vi "eFGV - Stop RT.vi"(6 "State":T1, 8 "error in (no error)":errorcluster, 10 "Stop RT":bool) -> (0 "error out":errorcluster, 2 "Stop RT Event":refnum<user-event>)   [LabVIEW 2020]
uses:
  Shared/Control/State - eFGV.ctl
  <vilib>/event_ctls.llb/usereventprio.ctl
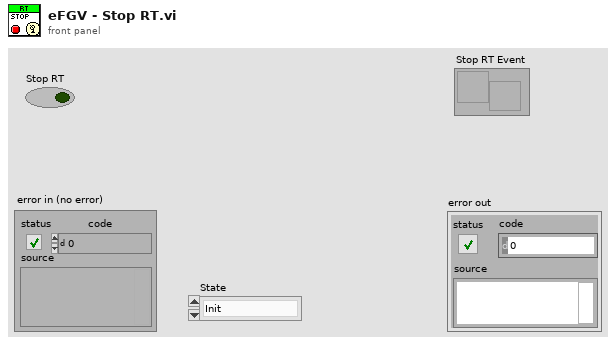
[diagram p1: front panel]
types:
  T1 = typedef "State - eFGV.ctl" = enum16{"Init", "Read", "Write", "Close"}
  T2 = typedef "usereventprio.ctl" = enum32{"high priority", "normal priority"}
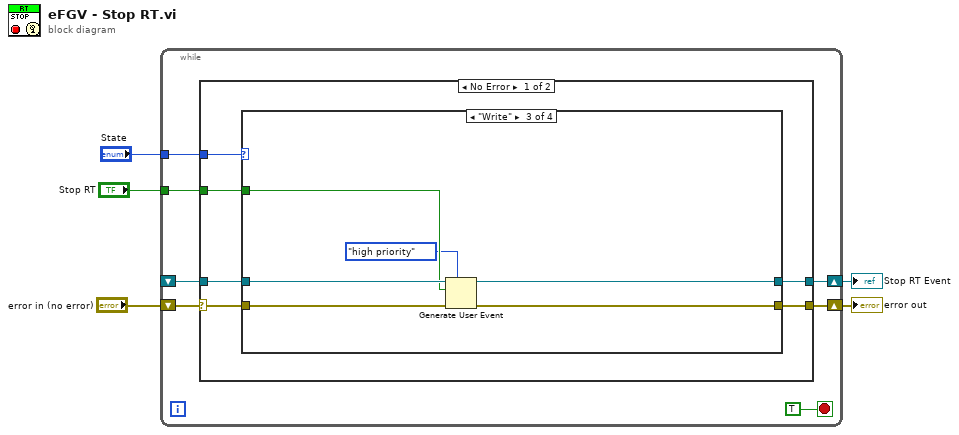
[diagram p0: block diagram]
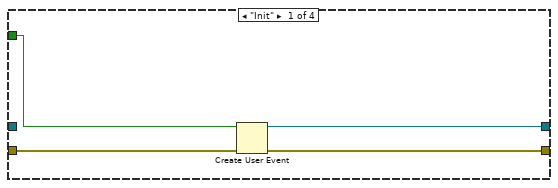
[diagram p2: hidden frame]
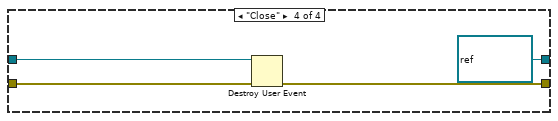
[diagram p4: hidden frame]
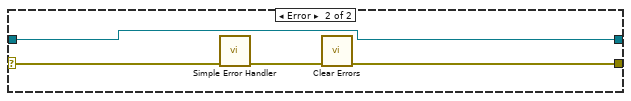
[diagram p5: hidden frame]
diagram:
  n1 = while {
    tunnel: "State" -> [w11]
    shift-right: [w9] -> w2
    shift-left: "error in (no error)" -> [w10]
    tunnel: "Stop RT" -> [w8]
    shift-right: [w7] -> w1
    shift-left: _ -> [w6]
    stop <- TRUE stop-if-true
    n2 = case shown="No Error" w10 {
      selector: w10 -> [w17 w38]
      tunnel: w11 -> [w18 _]
      tunnel: [w16 w36] -> w9
      tunnel: w8 -> [w15 _]
      tunnel: [w14 w35] -> w7
      tunnel: w6 -> [w13 w35]
      frame No Error {
        n3 = case shown="\"Write\"" w18 {
          tunnel: w17 -> [w22 w24 w30 w34]
          tunnel: [w21 w24 w29 w33] -> w16
          tunnel: w15 -> [w20 _ w27 _]
          tunnel: [w19 w23 w26 refnum<user-event> refnum ("Stop RT")] -> w14
          tunnel: w13 -> [_ w23 w28 w32]
          frame "Init" {
            n4 = Create User Event(user event datatype=w20, error in=w22) -> (user event=w19:refnum<user-event>, error out=w21:errorcluster)
          }
          frame "Read", Default {
          }
          frame "Write" {
            n5 = Generate User Event(priority (normal)=usereventprio."high priority", user event=w28, event data cluster=w27, error in=w30) -> (user event out=w26:refnum<user-event>, error out=w29:errorcluster)
          }
          frame "Close" {
            n6 = Destroy User Event(user event=w32, error in=w34) -> (error out=w33:errorcluster)
          }
        }
      }
      frame Error {
        n7 = call <vilib>:"Simple Error Handler.vi"("error in (no error)"=w38) -> ("error out"=w37:errorcluster)  [unwired: 4 in, 4 out]
        n8 = call <vilib>:"Clear Errors.vi"("error in (no error)"=w37) -> ("error out"=w36:errorcluster)  [unwired: 5 in, 1 out]
      }
    }
  }
  "error out" <- w2
  "Stop RT Event" <- w1
